vi "Register to Discovery Service.vi"(0 "gRPC ID in":T2, 5 "port number":i32, 7 "measurement plugin service in":refnum<class "Measurement Plugin Service.lvclass">, 9 "measurement service in":refnum<class "IMeasurement Service.lvclass">[](array[class]), 11 "error in":errorcluster) -> (4 "gRPC ID out":T2, 6 "response data":T1, 8 "measurement plugin service out":refnum<class "Measurement Plugin Service.lvclass">, 10 "measurement service out":refnum<class "IMeasurement Service.lvclass">[](array[class]), 15 "error out":errorcluster)   [LabVIEW 2020, in "Measurement Plugin Measurement Server.lvlib"]
uses:
  Measurement Plugin Measurement Server.lvlib
  gRPC/Generated APIs/ni/measurementlink/discovery/v1/ni.measurementlink.discovery.v1.lvlib
  gRPC/Generated APIs/ni/measurementlink/discovery/v1/RPC Messages/ni_measurementlink_discovery_v1_RegisterServiceRequest.ctl
  gRPC/Generated APIs/ni/measurementlink/discovery/v1/RPC Messages/ni_measurementlink_discovery_v1_ServiceLocation.ctl
  gRPC/Generated APIs/ni/measurementlink/discovery/v1/RPC Messages/ni_measurementlink_discovery_v1_ServiceDescriptor.ctl
  Measurement Plugin Service/Measurement Plugin Service.lvclass
  IMeasurement Service/IMeasurement Service.lvclass
  gRPC/Generated APIs/ni/measurementlink/discovery/v1/RPC Messages/ni_measurementlink_discovery_v1_ServiceDescriptor_AnnotationsEntry.ctl
  <vilib>/gRPC/LabVIEW gRPC Library/Shared/grpcId.ctl
  <vilib>/gRPC/LabVIEW gRPC Library/grpc-lvsupport-release.lvlib
  gRPC/Generated APIs/ni/measurementlink/discovery/v1/RPC Messages/ni_measurementlink_discovery_v1_RegisterServiceResponse.ctl
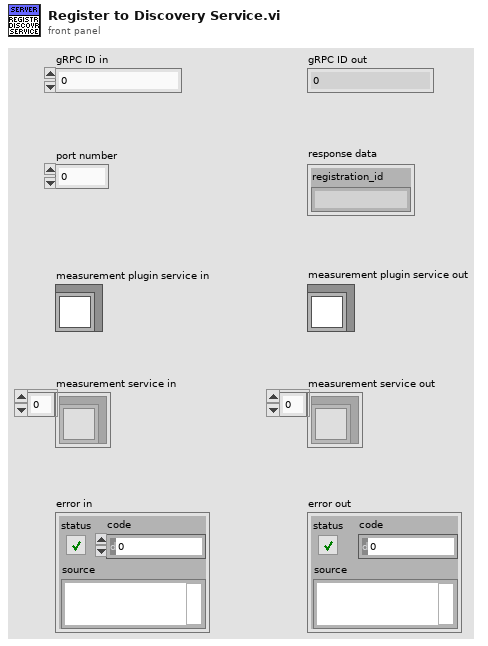
[diagram p1: front panel]
types:
  T1 = typedef "ni.measurementlink.discovery.v1.lvlib/ni_measurementlink_discovery_v1_RegisterServiceResponse.ctl" = cluster{"registration_id":string}
  T2 = typedef "grpc-lvsupport-release.lvlib/grpcId.ctl" = u64
  T3 = typedef "ni.measurementlink.discovery.v1.lvlib/ni_measurementlink_discovery_v1_RegisterServiceRequest.ctl" = cluster{"service_description":T4, "location":T6}
  T4 = typedef "ni.measurementlink.discovery.v1.lvlib/ni_measurementlink_discovery_v1_ServiceDescriptor.ctl" = cluster{"display_name":string, "description_url":string, "provided_interfaces":string[], "service_class":string, "annotations":T5[]}
  T5 = typedef "ni.measurementlink.discovery.v1.lvlib/ni_measurementlink_discovery_v1_ServiceDescriptor_AnnotationsEntry.ctl" = cluster{"key":string, "value":string}
  T6 = typedef "ni.measurementlink.discovery.v1.lvlib/ni_measurementlink_discovery_v1_ServiceLocation.ctl" = cluster{"location":string, "insecure_port":string, "ssl_authenticated_port":string}
  T7 = typedef "Measurement Plugin Measurement Server.lvlib/Measurement Details.ctl" = cluster{"display name":string, "version":string}
  T8 = typedef "Measurement Plugin Measurement Server.lvlib/Measurement Annotation.ctl" = cluster{"key":string, "value":string}
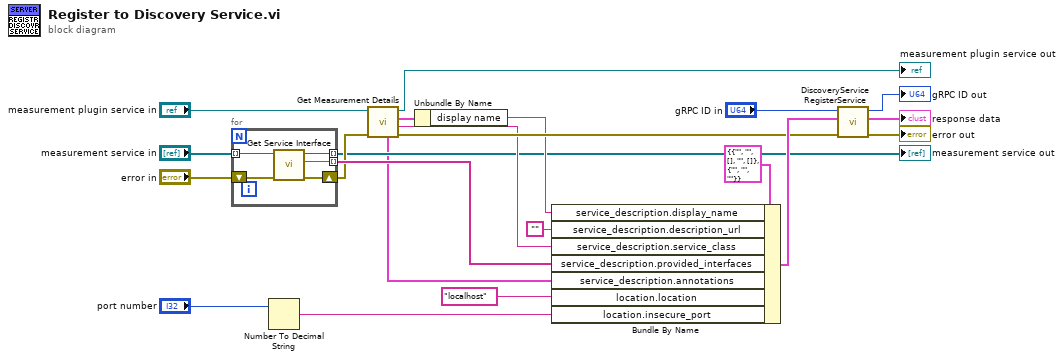
[diagram p0: block diagram]
diagram:
  n1 = for {
    tunnel: "measurement service in" -> [w27] mode=indexing
    tunnel: [w26] -> w7 mode=indexing
    shift-right: [w24] -> w5
    shift-left: "error in" -> [w25]
    tunnel: [w23] -> w3 mode=indexing
    n2 = call-dynamic "Get Service Interface.vi"("error in"=w25, "measurement service in"=w27) -> ("error out"=w24:errorcluster, "service interface"=w26:string, "measurement service out"=w23:refnum<class "IMeasurement Service.lvclass">)  [unwired: 7 in]
  }
  "measurement service out" <- w3
  n3 = Number To Decimal String(number="port number") -> (decimal integer string=w22:string)  [unwired: 1 in]
  n4 = call-dynamic "Get Measurement Details.vi"("error in"=w5, "measurement plugin service in"="measurement plugin service in") -> ("error out"=w11:errorcluster, "service class"=w9:string, "measurement details"=w10:T7, "measurement plugin service out"=→"measurement plugin service out":refnum<class "Measurement Plugin Service.lvclass">, "measurement annotations"=w1:T8[])  [unwired: 5 in]
  n5 = Unbundle By Name(w10) -> ("display name"=w8:string)
  n6 = Bundle By Name(cluster=T3 {"service_description"={"display_name"="", "description_url"="", "provided_interfaces"=[], "service_class"="", "annotations"=[]}, "location"={"location"="", "insecure_port"="", "ssl_authenticated_port"=""}} ("Request Data"), "service_description.display_name"=w8, "service_description.description_url"="", "service_description.service_class"=w9, "service_description.provided_interfaces"=w7, "service_description.annotations"=w1, "location.location"="localhost", "location.insecure_port"=w22) -> (w17:T3)
  n7 = call "DiscoveryService RegisterService.vi"("error in"=w11, "Request Data"=w17, "gRPC ID"="gRPC ID in") -> ("error out"=→"error out":errorcluster, "Response Data"=→"response data":T1, "gRPC ID out"=→"gRPC ID out":T2)  [unwired: 6 in]
